vi "Loop bar Status.vi"() -> ()   [LabVIEW 2015]
panel:
  out "Loop status bar":T1 {"loop in progress" scale=0.0..100.0}
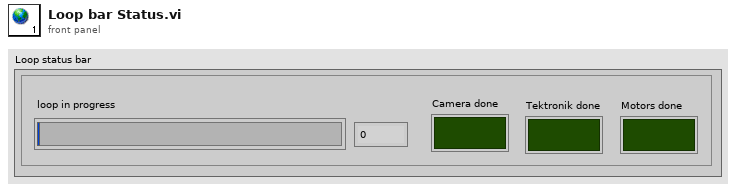
[diagram p1: front panel]
types:
  T1 = cluster{"Camera done":bool, "Tektronik done":bool, "Motors done":bool, "loop in progress":u8}
diagram:
